vi "Queue Caller.vi"(9 "Priority?":bool, 10 "Msg":refnum<class "Msg.lvclass">, 11 "Base Event Actor in":refnum<class "Base Event Actor.lvclass">) -> (3 "Base Event Actor out":refnum<class "Base Event Actor.lvclass">)   [LabVIEW 2021, in "jettl.lvlib" / "Base Event Actor.lvclass"]
uses:
  Base Event Actor.lvclass
  Msg/Msg/Msg.lvclass
  Base Event Actor.lvclass/Base Event Actor.ctl
  jettl.lvlib
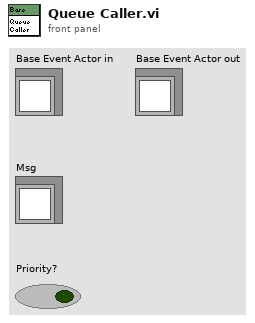
[diagram p1: front panel]
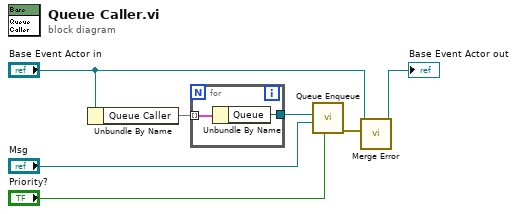
[diagram p0: block diagram]
diagram:
  n1 = Unbundle By Name("Base Event Actor in") -> ("Queue Caller"=w6:map{string, refnum<data-value>})
  n2 = for {
    tunnel: [w8] -> w5
    tunnel: w6 -> [w9] mode=indexing
    n3 = Unbundle By Name(w9) -> ("Queue"=w8:refnum<data-value>)
  }
  n4 = call "Queue Enqueue.vi"("Priority?"="Priority?", "Msg"="Msg", "Queue"=w5) -> ("error out"=w7:errorcluster)  [unwired: 8 in]
  n5 = call-dynamic "Merge Error.vi"("Error"=w7, "Base Event Actor in"="Base Event Actor in") -> ("Base Event Actor out"=→"Base Event Actor out":refnum<class "Base Event Actor.lvclass">)  [unwired: 9 in]
